vi "Lab 2 Q2.vi"() -> ()   [LabVIEW 2016]
panel:
  out "Meter":i32(knob) scale=0.0..10.0
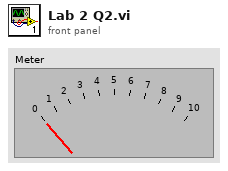
[diagram p1: front panel]
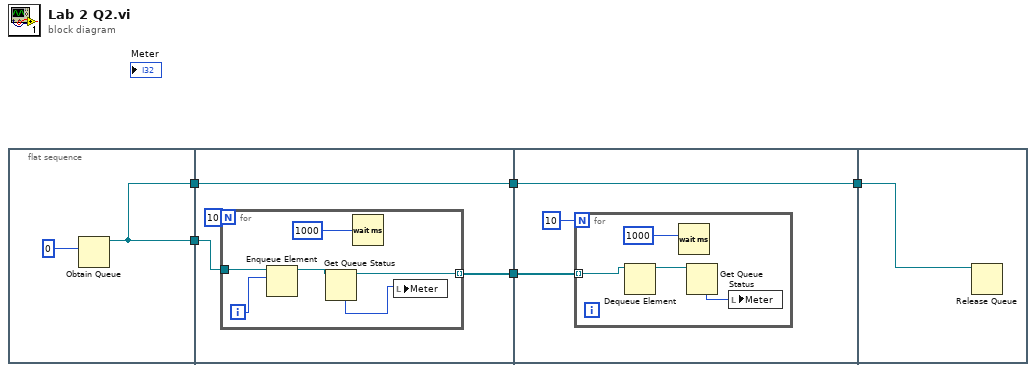
[diagram p0: block diagram]
diagram:
  n1 = flat-sequence {
    tunnel: [w7] -> w5
    tunnel: [w7] -> w3
    tunnel: w5 -> [w10]
    tunnel: [w9] -> w4
    tunnel: w3 -> [w8]
    tunnel: [w8] -> w2
    tunnel: w4 -> [w19]
    tunnel: w2 -> [w18]
    tunnel: [w18] -> w1
    tunnel: w1 -> [w25]
    frame #0 {
      n2 = Obtain Queue(element data type=0) -> (queue out=w7:refnum<queue>)  [unwired: 4 in, 2 out]
    }
    frame #1 {
      n3 = for {
        N: 10 -> [_]
        tunnel: w10 -> [w17]
        tunnel: [w13] -> w9 mode=indexing
        i -> [w16]
        n4 = Enqueue Element(queue=w17, element=w16) -> (queue out=w14:refnum<queue>)  [unwired: 2 in, 2 out]
        n5 = Get Queue Status(queue=w14) -> (queue out=w13:refnum<queue>, # elements in queue=w15:i32)  [unwired: 2 in, 6 out]
        n6 = Wait (ms)(milliseconds to wait=u32 1000) -> ()  [unwired: 1 out]
        n7 = local write "Meter"(w15) -> ()
      }
    }
    frame #2 {
      n8 = for {
        N: 10 -> [_]
        tunnel: w19 -> [w24] mode=indexing
        n9 = Dequeue Element(queue=w24) -> (queue out=w23:refnum<queue>)  [unwired: 2 in, 3 out]
        n10 = Wait (ms)(milliseconds to wait=u32 1000) -> ()  [unwired: 1 out]
        n11 = Get Queue Status(queue=w23) -> (# elements in queue=w22:i32)  [unwired: 2 in, 7 out]
        n12 = local write "Meter"(w22) -> ()
      }
    }
    frame #3 {
      n13 = Release Queue(queue=w25) -> ()  [unwired: 2 in, 3 out]
    }
  }
